vi "Filter_Array.vi"() -> ()   [LabVIEW 2016]
panel:
  out "Result":dbl[](array[numeric]) format="%.2f"
  in  "2D array":dbl[][](array[numeric]) format="%.2f"
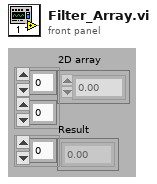
[diagram p1: front panel]
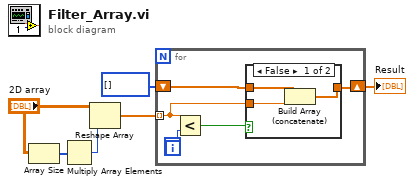
[diagram p0: block diagram]
diagram:
  n1 = Array Size(array="2D array") -> (size(s)=w5:i32[])
  n2 = Multiply Array Elements(1:w5) -> (0:w4:i32)
  n3 = Reshape Array("2D array", w4) -> (w3:dbl[])
  n4 = for {
    tunnel: w3 -> [w9] mode=indexing
    shift-right: [w7] -> w1
    shift-left: i32[] [] ("Constante tableau") -> [w8]
    n5 = Less?(x=w9, y=10) -> (x < y?=w10:bool)
    n6 = case shown="False" w10 {
      tunnel: w9 -> [w13 _]
      tunnel: w8 -> [w14 w15]
      tunnel: [w12 w15] -> w7
      frame False {
        n7 = Build Array (concatenate)(w14, w13) -> (w12:dbl[])
      }
      frame True {
      }
    }
  }
  "Result" <- w1
